vi "Update UI per Reference.vi"(8 "error in (no error)":errorcluster, 11 "Analyze Results q-Factor in":refnum<class "Analyze Results q-Factor.lvclass">) -> (0 "error out":errorcluster, 3 "Analyze Results q-Factor out":refnum<class "Analyze Results q-Factor.lvclass">)   [LabVIEW 2020, in "Analyze Results q-Factor.lvclass"]
uses:
  Analyze Results q-Factor.lvclass
  Analyze Results q-Factor.lvclass/Analyze Results q-Factor.ctl
  Results Base/Analyze Results Base.lvclass
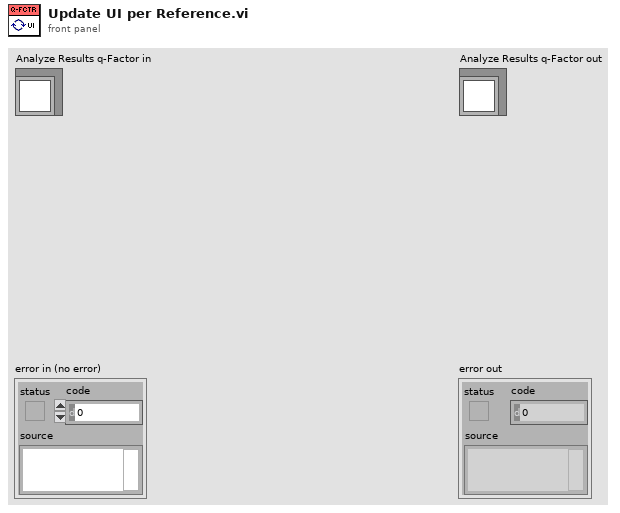
[diagram p1: front panel]
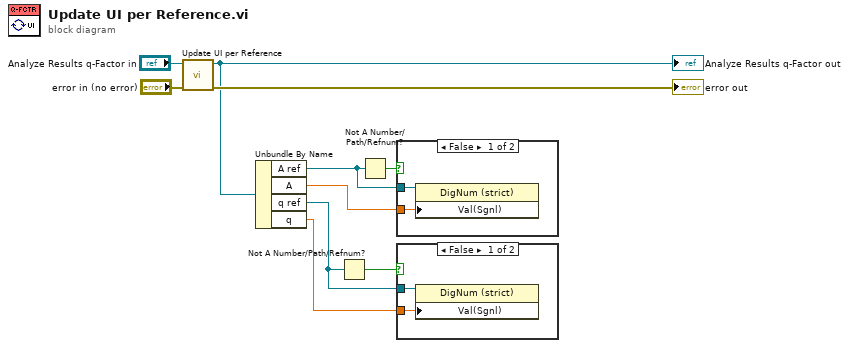
[diagram p0: block diagram]
diagram:
  n1 = call-parent "Update UI per Reference.vi"("error in (no error)"="error in (no error)", "Analyze Results Base in"="Analyze Results q-Factor in") -> ("error out"=→"error out":errorcluster, "Analyze Results Base out"=w7:refnum<class "Analyze Results q-Factor.lvclass">)  [unwired: 8 in]
  "Analyze Results q-Factor out" <- w7
  n2 = Unbundle By Name(w7) -> ("A ref"=w4:refnum<vi>, "A"=w3:dbl[unit], "q ref"=w2:refnum<vi>, "q"=w1:dbl)
  n3 = Not A Number/Path/Refnum?(number/path/refnum=w2) -> (NaN/Path/Refnum?=w6:bool)
  n4 = Not A Number/Path/Refnum?(number/path/refnum=w4) -> (NaN/Path/Refnum?=w5:bool)
  n5 = case shown="False" w5 {
    tunnel: w4 -> [w12 _]
    tunnel: w3 -> [w11 _]
    frame False {
      n6 = property class="DigNum (strict)"(reference=w12, "Val(Sgnl)"=w11) -> ()  [unwired: 1 in, 2 out]
    }
    frame True {
    }
  }
  n7 = case shown="False" w6 {
    tunnel: w2 -> [w14 _]
    tunnel: w1 -> [w13 _]
    frame False {
      n8 = property class="DigNum (strict)"(reference=w14, "Val(Sgnl)"=w13) -> ()  [unwired: 1 in, 2 out]
    }
    frame True {
    }
  }
